vi "toNextHour.vi"(11 "Cron in":T1) -> (3 "Cron out":T1)   [LabVIEW 2013, in "openCron.lvlib" / "Cron.lvclass"]
uses:
  Cron.lvclass
  CronTime -- cluster.ctl
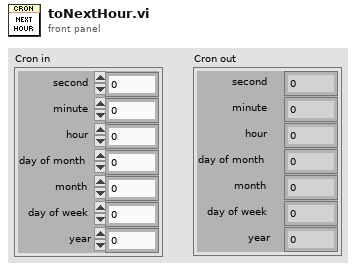
[diagram p1: front panel]
types:
  T1 = typedef "openCron.lvlib/Cron.lvclass/CronTime -- cluster.ctl" = cluster{"second":i32, "minute":i32, "hour":i32, "day of month":i32, "month":i32, "day of week":i32, "year":i32}
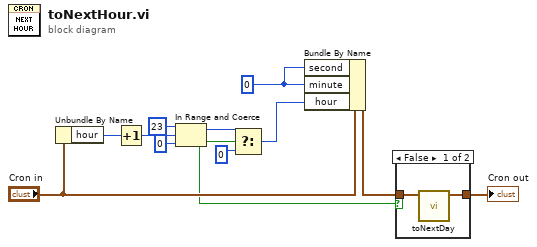
[diagram p0: block diagram]
diagram:
  w5 = 0 ("hour")
  n1 = Unbundle By Name("Cron in") -> ("hour"=w12:i32)
  n2 = Increment(x=w12) -> (x+1=w10:i32)
  n3 = In Range and Coerce(upper limit=23, x=w10, lower limit=0) -> (coerced(x)=w8:i32, In Range?=w2:bool)
  n4 = Select(t=w8, s=w2, f=0 ("month")) -> (s? t:f=w1:i32)
  n5 = Bundle By Name(cluster="Cron in", "second"=w5, "minute"=w5, "hour"=w1) -> (w4:T1)
  n6 = case shown="False" w2 {
    tunnel: w4 -> [w14 w15]
    tunnel: [w13 w15] -> w3
    frame False {
      n7 = call "toNextDay.vi"("Cron in"=w14) -> ("Cron out"=w13:T1)  [unwired: 10 in]
    }
    frame True {
    }
  }
  "Cron out" <- w3
